vi "joystickScale.vi"(1 "Logarithmic?":bool, 2 "joystick in":dbl, 3 "max":dbl, 4 "min":dbl) -> (0 "joystick out":dbl)   [LabVIEW 2012]
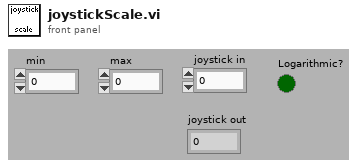
[diagram p1: front panel]
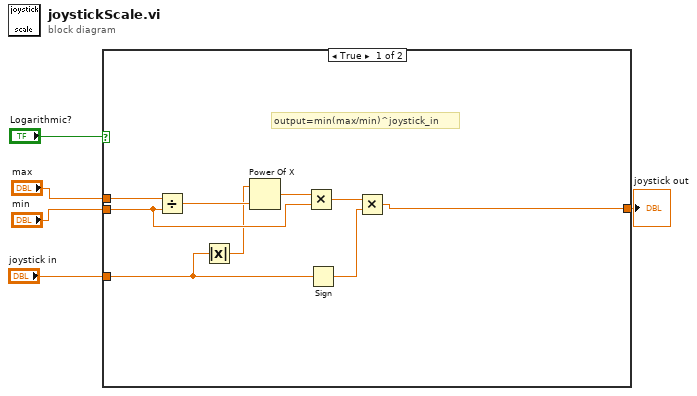
[diagram p0: block diagram]
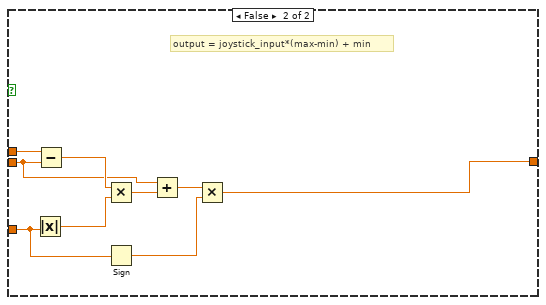
[diagram p2: hidden frame]
diagram:
  n1 = case shown="True" "Logarithmic?" {
    tunnel: "min" -> [w11 w19]
    tunnel: "max" -> [w14 w23]
    tunnel: "joystick in" -> [w7 w17]
    tunnel: [w8 w15] -> w1
    frame True {
      # "output=min(max/min)^joystick_in"
      n2 = Divide(x=w14, y=w11) -> (x/y=w13:dbl)
      n3 = Absolute Value(x=w7) -> (abs(x)=w6:dbl)
      n4 = Power Of X(1:w13, 2:w6) -> (0:w12:dbl)
      n5 = Multiply(x=w12, y=w11) -> (x*y=w10:dbl)
      n6 = Sign(1:w7) -> (0:w9:dbl)
      n7 = Multiply(x=w10, y=w9) -> (x*y=w8:dbl)
    }
    frame False {
      # "output = joystick_input*(max-min) + min"
      n8 = Absolute Value(x=w17) -> (abs(x)=w22:dbl)
      n9 = Subtract(x=w23, y=w19) -> (x-y=w21:dbl)
      n10 = Multiply(x=w21, y=w22) -> (x*y=w20:dbl)
      n11 = Sign(1:w17) -> (0:w16:dbl)
      n12 = Add(x=w19, y=w20) -> (x+y=w18:dbl)
      n13 = Multiply(x=w18, y=w16) -> (x*y=w15:dbl)
    }
  }
  "joystick out" <- w1
